vi "Outside Fan PWM Control.vi"() -> ()   [LabVIEW 2020]
uses:
  type defs/Source_Destination.ctl
  type defs/ERD Write Data In.ctl
  type defs/Data Type.ctl
  library/GEA2_Toolkit.lvlib
panel:
  out "Counter":i32
  in  "Number of Cycles":i32=5
  in  "PWM Value 2":i32
  in  "PWM Value":i32
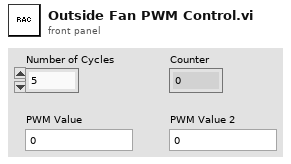
[diagram p1: front panel]
types:
  T1 = typedef "GEA2_Toolkit.lvlib/ERD Write Data In.ctl" = cluster{"ERD Number":u16, "Data Type":T2, "Data":string}
  T2 = typedef "GEA2_Toolkit.lvlib/Data Type.ctl" = enum16{"string", "boolean", "uint8_t", "uint16_t", "uint32_t", "uint64_t", "int8_t", "int16_t", "int32_t", "int64_t"}
  T3 = typedef "GEA2_Toolkit.lvlib/Source_Destination.ctl" = cluster{"Source":u8, "Destination":u8}
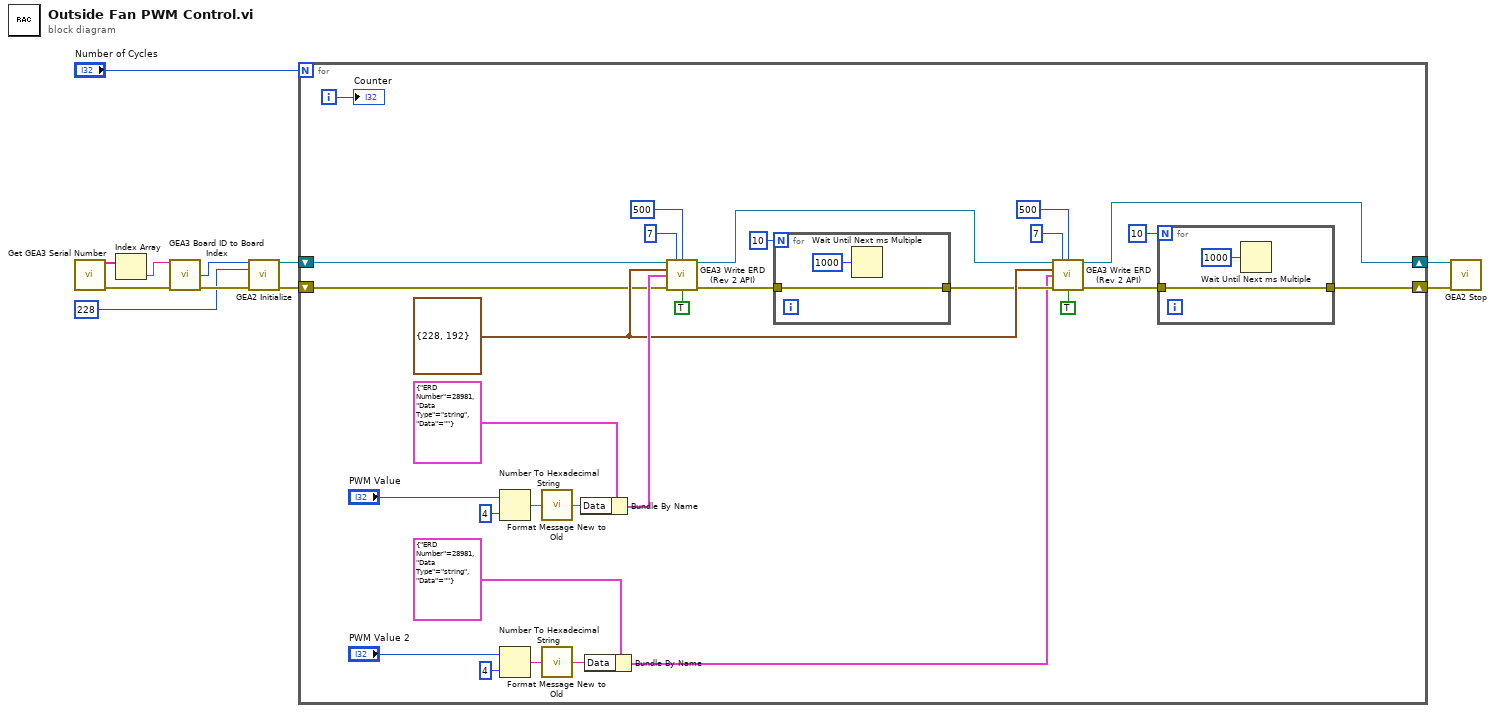
[diagram p0: block diagram]
diagram:
  n1 = call "Get GEA3 Serial Number.vi"() -> ("GEA3 Serial Numbers"=w6:string[], "Error Out"=w7:errorcluster)  [unwired: 14 in]
  n2 = Index Array(array=w6) -> (element=w5:string)  [unwired: 1 in]
  n3 = call "GEA3 Board ID to Board Index.vi"("GEA3 Serial Number"=w5, "Error In"=w7) -> ("Board Index"=w8:i32, "Error Out"=w9:errorcluster)  [unwired: 9 in, 3 out]
  n4 = call "GEA2 Initialize.vi"("Board Index"=w8, "Source Address"=u8 228, "error in"=w9) -> ("GEA2 Reference Out"=w3:refnum<k24>, "error out"=w2:errorcluster)  [unwired: 10 in, 1 out]
  n5 = for {
    N: "Number of Cycles" -> [_]
    shift-right: [w18] -> w11
    shift-left: w3 -> [w17]
    shift-right: [w13] -> w10
    shift-left: w2 -> [w16]
    i -> [w12]
    w26 = T3 {"Source"=228, "Destination"=192} ("GEA Inputs")
    n6 = Number To Hexadecimal String(1:i16 4 ("width (-)"), 2:"PWM Value") -> (0:w39:string)
    n7 = Number To Hexadecimal String(1:i16 4 ("width (-)"), 2:"PWM Value 2") -> (0:w21:string)
    n8 = call "Format Message New to Old.vi"("Raw Message In"=w39) -> ("Conv Message Out"=w35:string)  [unwired: 14 in]
    n9 = call "Format Message New to Old.vi"("Raw Message In"=w21) -> ("Conv Message Out"=w24:string)  [unwired: 14 in]
    n10 = Bundle By Name(cluster=T1 {"ERD Number"=28981, "Data Type"=enum."string", "Data"=""} ("ERD Write Data In"), "Data"=w35) -> (w36:T1)
    n11 = Bundle By Name(cluster=T1 {"ERD Number"=28981, "Data Type"=enum."string", "Data"=""} ("ERD Write Data In"), "Data"=w24) -> (w19:T1)
    n12 = call "GEA3 Write ERD (Rev 2 API).vi"("GEA2 Reference In"=w17, "# of Tries"=u8 7, "Read Timeout (ms)"=u32 500, "GEA Inputs"=w26, "ERD Write Data In"=w36, "Error In"=w16, "Verify ERD Response?"=TRUE) -> ("GEA2 Reference Out"=w27:refnum<k24>, "Error Out"=w32:errorcluster)  [unwired: 5 in, 2 out]
    n13 = for {
      N: 10 -> [_]
      tunnel: w32 -> [w45]
      tunnel: [w45] -> w25
      n14 = Wait Until Next ms Multiple(millisecond multiple=u32 1000) -> ()  [unwired: 1 out]
    }
    n15 = call "GEA3 Write ERD (Rev 2 API).vi"("GEA2 Reference In"=w27, "# of Tries"=u8 7, "Read Timeout (ms)"=u32 500, "GEA Inputs"=w26, "ERD Write Data In"=w19, "Error In"=w25, "Verify ERD Response?"=TRUE) -> ("GEA2 Reference Out"=w18:refnum<k24>, "Error Out"=w14:errorcluster)  [unwired: 5 in, 2 out]
    n16 = for {
      N: 10 -> [_]
      tunnel: w14 -> [w43]
      tunnel: [w43] -> w13
      n17 = Wait Until Next ms Multiple(millisecond multiple=u32 1000) -> ()  [unwired: 1 out]
    }
    "Counter" <- w12
  }
  n18 = call "GEA2 Stop.vi"("GEA2 Reference In"=w11, "Error In"=w10) -> ()  [unwired: 13 in, 1 out]
